vi "dfd_DFXPSimu Casting (scaler).vi"(5 "quantize output? (T)":bool=TRUE, 7 "op params":T2={"source"=0, "is floating?"=FALSE, "o-mode"=enum."Wrap", "q-mode"=enum."Truncation", "wl"=1, "high limit"=0, "low limit"=0, "iwl"=0, "sign?"=TRUE} {"source" items=["Coef a/k"=0, "Coef b/v"=7, "Input"=1, "Output"=2, "Multiplicand"=3, "Product"=4, "Sum"=5, "Delay"=6, "Gain"=8]}, 8 "filtering statistics in":T6(array[cluster]) {"statistics information"."min value" format="%.2f"; "statistics information"."max value" format="%.2f"; "Quantizer Source" items=["Coefficients a/k"=0, "Coefficients b/v"=7, "Input"=1, "Output"=2, "Multiplicand"=3, "Product"=4, "Sum"=5, "Delay"=6]}, 11 "Value in":T7 {"Low 64" format="%.0x"; "High 64" format="%.0x"}) -> (0 "filtering statistics out":T6(array[cluster]) {"statistics information"."min value" format="%.2f"; "statistics information"."max value" format="%.2f"; "Quantizer Source" items=["Coefficients a/k"=0, "Coefficients b/v"=7, "Input"=1, "Output"=2, "Multiplicand"=3, "Product"=4, "Sum"=5, "Delay"=6]}, 3 "Value out":T1={"value"=0, "wl"=0, "iwl"=0, "Signed"=TRUE} {"value" format="%.0x"})   [LabVIEW 2017, in "NI_DigFilter_FXP.lvlib"]
uses:
  <vilib>/addons/Digital Filter Design/NI_DigFilter_FXP.lvlib
  <vilib>/addons/Digital Filter Design/_Objects.llb/dfd_DFXP Data Type 128bits (scaler).ctl
  <vilib>/addons/Digital Filter Design/_Objects.llb/dfd_DFXP Data Type (scaler).ctl
  <vilib>/addons/Digital Filter Design/_Objects.llb/DFD Quantization Sources.ctl
  <vilib>/addons/Digital Filter Design/_Objects.llb/DFD FXP Statistics Data.ctl
  <vilib>/addons/Digital Filter Design/_Objects.llb/dfd_DFXP Operation Parameter.ctl
  <vilib>/addons/Digital Filter Design/_Objects.llb/dfd_Internal Quantization Srcs.ctl
  <vilib>/addons/Digital Filter Design/NI_DigFilterLicensed.lvlib
panel:
  in  "Value out type":T1={"value"=0, "wl"=0, "iwl"=0, "Signed"=TRUE} {"value" format="%.0x"}
  in  "Value out type":T1={"value"=0, "wl"=0, "iwl"=0, "Signed"=TRUE} {"value" format="%.0x"}
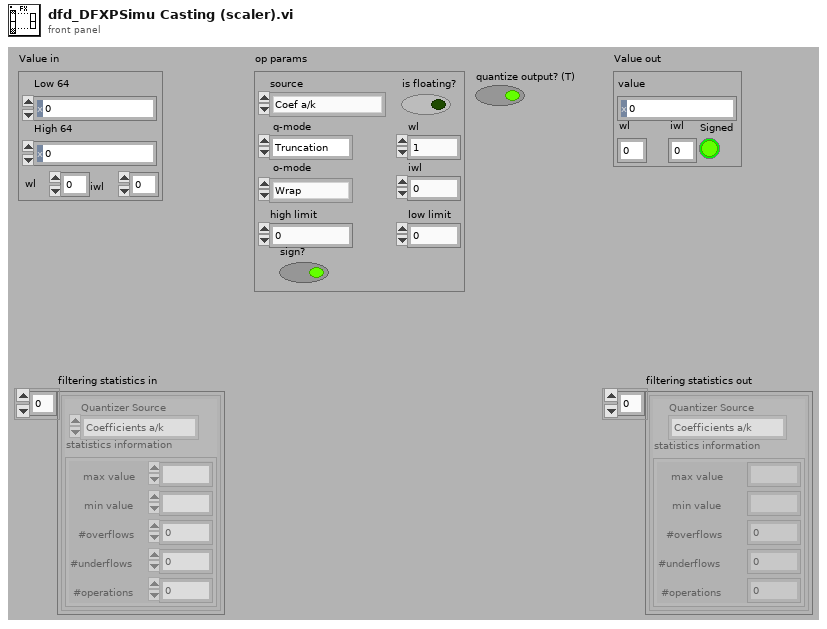
[diagram p1: front panel]
types:
  T1 = typedef "dfd_DFXP Data Type (scaler).ctl" = cluster{"value":i64, "wl":i16, "iwl":i16, "Signed":bool}
  T2 = typedef "dfd_DFXP Operation Parameter.ctl" = cluster{"source":T3, "is floating?":bool, "o-mode":enum16{"Saturation", "Wrap"}, "q-mode":enum16{"Nearest", "Truncation"}, "wl":i16, "high limit":i64, "low limit":i64, "iwl":i16, "sign?":bool}
  T3 = typedef "NI_DigFilterLicensed.lvlib/dfd_Internal Quantization Srcs.ctl" = u16
  T4 = typedef "NI_DigFilterLicensed.lvlib/DFD Quantization Sources.ctl" = u16
  T5 = typedef "NI_DigFilterLicensed.lvlib/DFD FXP Statistics Data.ctl" = cluster{"max value":ext, "min value":ext, "#overflows":i32, "#underflows":i32, "#operations":i32}
  T6 = cluster{"Quantizer Source":T4, "statistics information":T5}[]
  T7 = typedef "dfd_DFXP Data Type 128bits (scaler).ctl" = cluster{"Low 64":u64, "High 64":i64, "wl":i16, "iwl":i16}
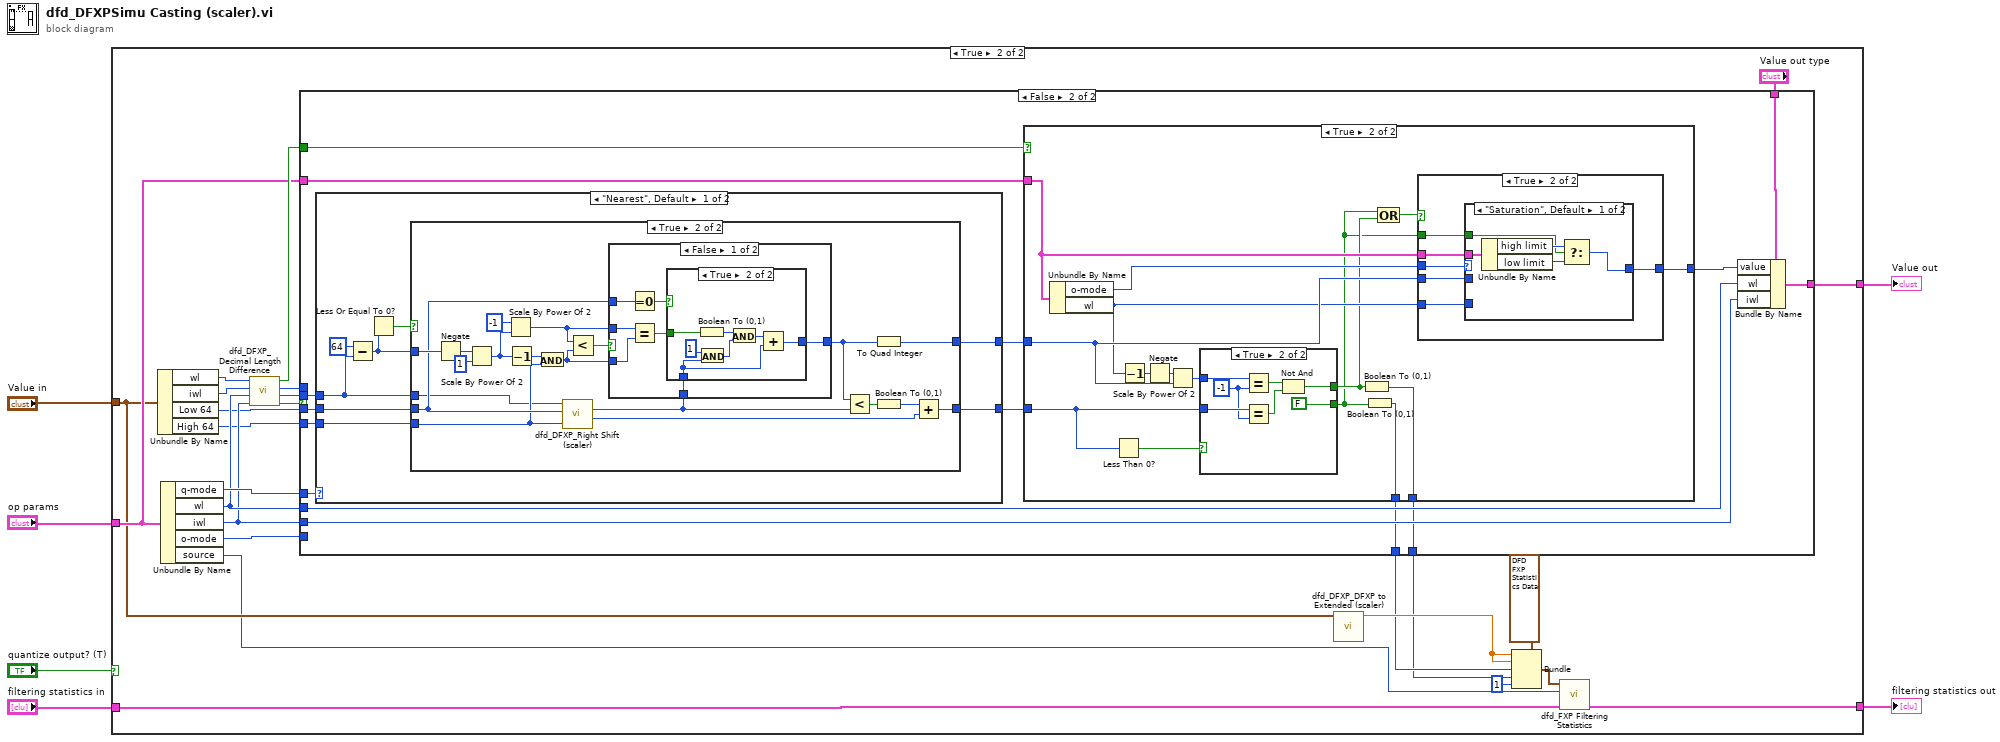
[diagram p0: block diagram]
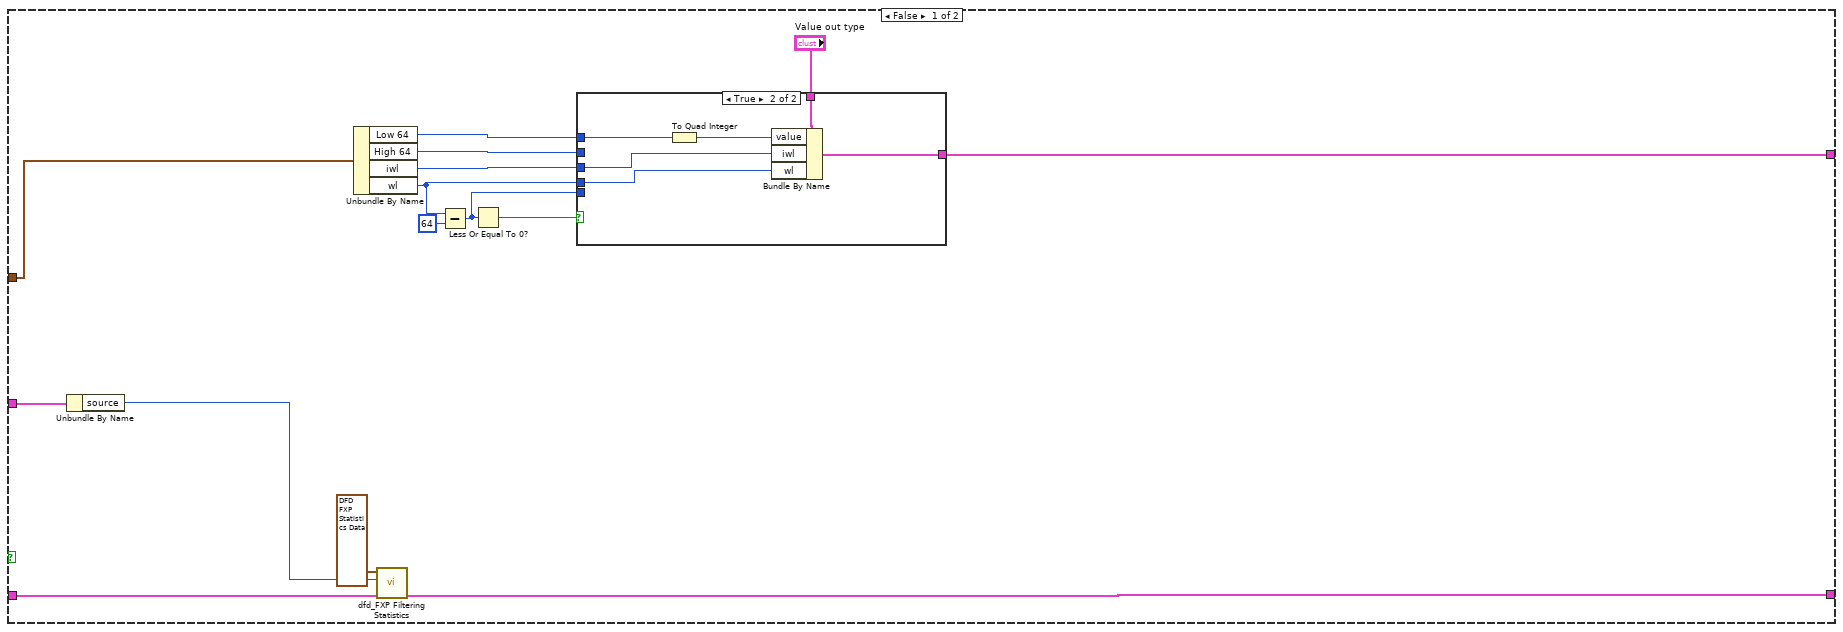
[diagram p2: hidden frame]
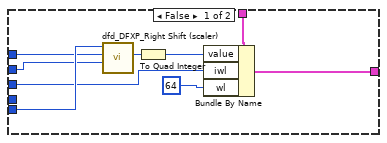
[diagram p3: hidden frame]
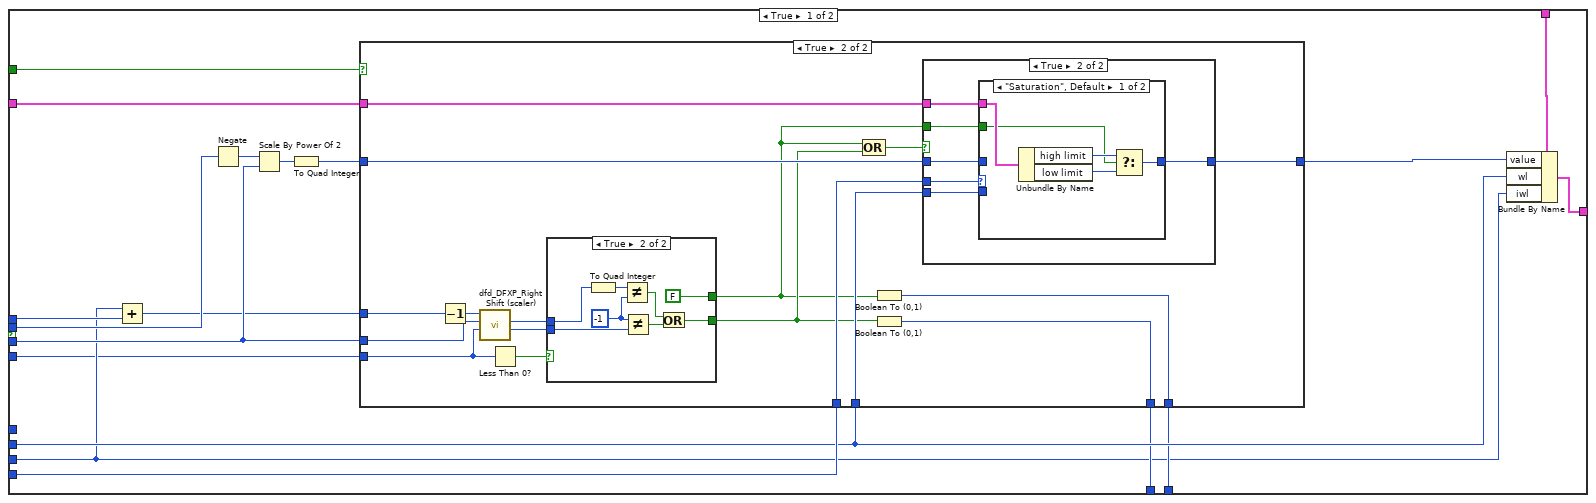
[diagram p4: hidden frame]
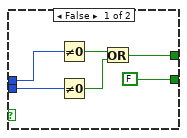
[diagram p6: hidden frame]
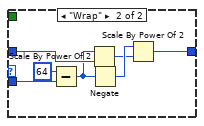
[diagram p8: hidden frame]
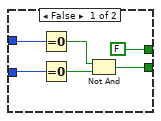
[diagram p10: hidden frame]
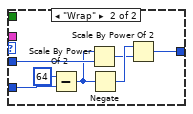
[diagram p12: hidden frame]
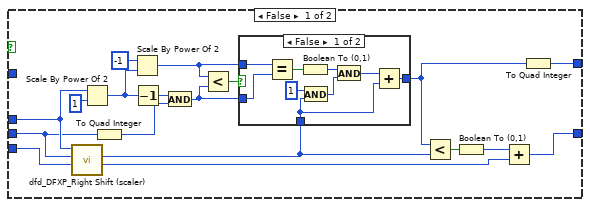
[diagram p13: hidden frame]
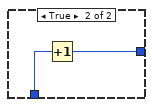
[diagram p14: hidden frame]
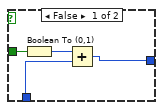
[diagram p15: hidden frame]
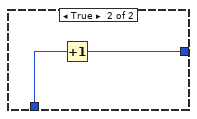
[diagram p16: hidden frame]
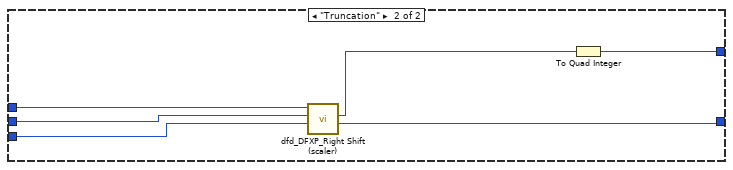
[diagram p17: hidden frame]
diagram:
  n1 = case shown="True" "quantize output? (T)" {
    tunnel: [w12 w50] -> w1
    tunnel: "op params" -> [w21 w53]
    tunnel: "Value in" -> [w13 w46]
    tunnel: "filtering statistics in" -> [w8 w39]
    tunnel: [w7 w38] -> w2
    frame False {
      n2 = Unbundle By Name(w21) -> ("source"=w10:T3)
      n3 = Unbundle By Name(w13) -> ("Low 64"=w19:u64, "High 64"=w17:i64, "iwl"=w18:i16, "wl"=w15:i16)
      n4 = call <vilib>:"dfd_FXP Filtering Statistics.vi"("filtering statistics in"=w8, "source"=w10, "new data"=T5 {"max value"=-inf, "min value"=inf, "#overflows"=0, "#underflows"=0, "#operations"=1}) -> ("filtering statistics out"=w7:T6)  [unwired: 8 in]
      n5 = Subtract(x=w15, y=i16 64) -> (x-y=w16:i16)
      n6 = Less Or Equal To 0?(x=w16) -> (x <= 0?=w11:bool)
      n7 = case shown="True" w11 {
        tunnel: w19 -> [w29 w36]
        tunnel: w18 -> [w25 w34]
        tunnel: [w23 w33] -> w12
        tunnel: w17 -> [w28 _]
        tunnel: w16 -> [w30 _]
        tunnel: w15 -> [_ w32]
        tunnel: "Value out type" -> [w22 w31]
        frame False {
          n8 = call <vilib>:"dfd_DFXP_Right Shift (scaler).vi"("High 64"=w28, "Low 64"=w29, "Num"=w30) -> ("Low 64"=w26:u64)  [unwired: 8 out]
          n9 = To Quad Integer(1:w26) -> (0:w27:i64)
          n10 = Bundle By Name(cluster=w22, "value"=w27, "iwl"=w25, "wl"=i16 64) -> (w23:T1)
        }
        frame True {
          n11 = To Quad Integer(1:w36) -> (0:w35:i64)
          n12 = Bundle By Name(cluster=w31, "value"=w35, "iwl"=w34, "wl"=w32) -> (w33:T1)
        }
      }
    }
    frame True {
      n13 = Unbundle By Name(w46) -> ("wl"=w59:i16, "iwl"=w60:i16, "Low 64"=w49:u64, "High 64"=w48:i64)
      n14 = Unbundle By Name(w53) -> ("q-mode"=w61:enum16{"Nearest", "Truncation"}, "wl"=w54:i16, "iwl"=w52:i16, "o-mode"=w55:enum16{"Saturation", "Wrap"}, "source"=w40:T3)
      n15 = call <vilib>:"dfd_DFXP_Decimal Length Difference.vi"("iwl 2"=w52, "wl 2"=w54, "iwl 1"=w60, "wl 1"=w59) -> ("fwl_diff <= 0?"=w58:bool, "fwl_diff"=w56:i16, "fwl"=w47:i16, "iwl_diff >= 0?"=w57:bool)  [unwired: 4 out]
      n16 = case shown="False" w58 {
        tunnel: w61 -> [_ w145]
        tunnel: w49 -> [w70 w144]
        tunnel: w53 -> [w78 w140]
        tunnel: w57 -> [w71 w142]
        tunnel: w56 -> [w69 w141]
        tunnel: w55 -> [w77 _]
        tunnel: w54 -> [w73 w137]
        tunnel: [w72 w135] -> w50
        tunnel: w52 -> [w64 w136]
        tunnel: "Value out type" -> [w75 w139]
        tunnel: [w68 w134] -> w43
        tunnel: [w67 w133] -> w42
        tunnel: w48 -> [w62 w132]
        tunnel: w47 -> [w65 _]
        frame True {
          n17 = Add(x=w64, y=w65) -> (x+y=w63:i16)
          n18 = Negate(x=w69) -> (-x=w79:i16)
          n19 = Scale By Power Of 2(n=w79, x=w70) -> (x*2^n=w76:u64)
          n20 = To Quad Integer(1:w76) -> (0:w66:i64)
          n21 = case shown="True" w71 {
            tunnel: w78 -> [_ w96]
            tunnel: w77 -> [_ w95]
            tunnel: w66 -> [w80 w94]
            tunnel: [w80 w93] -> w74
            tunnel: w73 -> [_ w92]
            tunnel: w70 -> [_ w88]
            tunnel: [_ w90] -> w68
            tunnel: [_ w91] -> w67
            tunnel: w63 -> [_ w89]
            tunnel: w62 -> [_ w81]
            frame False {
            }
            frame True {
              n22 = Decrement(x=w89) -> (x-1=w85:i16)
              n23 = call <vilib>:"dfd_DFXP_Right Shift (scaler).vi"("High 64"=w81, "Low 64"=w88, "Num"=w85) -> ("High 64"=w86:i64, "Low 64"=w87:u64)  [unwired: 7 out]
              n24 = Less Than 0?(x=w81) -> (x < 0?=w84:bool)
              n25 = case shown="True" w84 {
                tunnel: [w100 FALSE] -> w82
                tunnel: [FALSE w111] -> w83
                tunnel: w87 -> [w102 w107]
                tunnel: w86 -> [w101 w106]
                frame False {
                  n26 = Not Equal To 0?(x=w102) -> (x != 0?=w99:bool)
                  n27 = Not Equal To 0?(x=w101) -> (x != 0?=w98:bool)
                  n28 = Or(x=w99, y=w98) -> (x .or. y?=w100:bool)
                }
                frame True {
                  w109 = i64 -1 ("y")
                  n29 = To Quad Integer(1:w107) -> (0:w105:i64)
                  n30 = Not Equal?(x=w105, y=w109) -> (x != y?=w110:bool)
                  n31 = Not Equal?(x=w109, y=w106) -> (x != y?=w108:bool)
                  n32 = Or(x=w110, y=w108) -> (x .or. y?=w111:bool)
                }
              }
              n33 = Compound Arithmetic op=OR(w82, w83) -> (w97:bool)
              n34 = Boolean To (0,1)(Boolean=w82) -> (0, 1=w91:i16)
              n35 = Boolean To (0,1)(Boolean=w83) -> (0, 1=w90:i16)
              n36 = case shown="True" w97 {
                tunnel: w95 -> [_ w118]
                tunnel: [w112 w117] -> w93
                tunnel: w92 -> [_ w116]
                tunnel: w94 -> [w112 w115]
                tunnel: w96 -> [_ w114]
                tunnel: w82 -> [_ w113]
                frame False {
                }
                frame True {
                  n37 = case shown="\"Saturation\", Default" w118 {
                    tunnel: [w120 w129] -> w117
                    tunnel: w116 -> [_ w130]
                    tunnel: w115 -> [_ w128]
                    tunnel: w114 -> [w123 _]
                    tunnel: w113 -> [w119 _]
                    frame "Saturation", Default {
                      n38 = Unbundle By Name(w123) -> ("high limit"=w122:i64, "low limit"=w121:i64)
                      n39 = Select(t=w122, s=w119, f=w121) -> (s? t:f=w120:i64)
                    }
                    frame "Wrap" {
                      n40 = Subtract(x=i16 64, y=w130) -> (x-y=w126:i16)
                      n41 = Scale By Power Of 2(n=w126, x=w128) -> (x*2^n=w124:i64)
                      n42 = Negate(x=w126) -> (-x=w125:i16)
                      n43 = Scale By Power Of 2(n=w125, x=w124) -> (x*2^n=w129:i64)
                    }
                  }
                }
              }
            }
          }
          n44 = Bundle By Name(cluster=w75, "value"=w74, "wl"=w73, "iwl"=w64) -> (w72:T1)
        }
        frame False {
          n45 = case shown="\"Nearest\", Default" w145 {
            tunnel: w141 -> [w199 w275]
            tunnel: w144 -> [w200 w274]
            tunnel: [w198 w270] -> w143
            tunnel: w132 -> [w197 w273]
            tunnel: [w194 w271] -> w131
            frame "Nearest", Default {
              n46 = Subtract(x=i16 64 ("y"), y=w199) -> (x-y=w195:i16)
              n47 = Less Or Equal To 0?(x=w195) -> (x <= 0?=w196:bool)
              n48 = case shown="True" w196 {
                tunnel: w200 -> [w211 w240]
                tunnel: w199 -> [w212 w238]
                tunnel: [w202 w231] -> w198
                tunnel: w197 -> [w210 w239]
                tunnel: w195 -> [_ w242]
                tunnel: [w204 w232] -> w194
                frame False {
                  n49 = call <vilib>:"dfd_DFXP_Right Shift (scaler).vi"("High 64"=w210, "Low 64"=w211, "Num"=w212) -> ("High 64"=w205:i64, "Low 64"=w208:u64)  [unwired: 7 out]
                  n50 = Scale By Power Of 2(n=w212, x=i64 1) -> (x*2^n=w216:i64)
                  n51 = To Quad Integer(1:w211) -> (0:w209:i64)
                  n52 = Scale By Power Of 2(n=-1, x=w216) -> (x*2^n=w217:i64)
                  n53 = Decrement(x=w216) -> (x-1=w214:i64)
                  n54 = And(x=w214, y=w209) -> (x .and. y?=w218:i64)
                  n55 = Less?(x=w217, y=w218) -> (x < y?=w219:bool)
                  n56 = case shown="False" w219 {
                    tunnel: w217 -> [w228 _]
                    tunnel: w218 -> [w227 _]
                    tunnel: w208 -> [w220 w230]
                    tunnel: [w222 w229] -> w203
                    frame False {
                      n57 = Equal?(x=w228, y=w227) -> (x = y?=w225:bool)
                      n58 = Boolean To (0,1)(Boolean=w225) -> (0, 1=w224:i16)
                      n59 = And(x=u64 1, y=w220) -> (x .and. y?=w223:u64)
                      n60 = And(x=w224, y=w223) -> (x .and. y?=w221:u64)
                      n61 = Add(x=w221, y=w220) -> (x+y=w222:u64)
                    }
                    frame True {
                      n62 = Increment(x=w230) -> (x+1=w229:u64)
                    }
                  }
                  n63 = Less?(x=w203, y=w208) -> (x < y?=w207:bool)
                  n64 = Boolean To (0,1)(Boolean=w207) -> (0, 1=w206:i16)
                  n65 = Add(x=w206, y=w205) -> (x+y=w204:i64)
                  n66 = To Quad Integer(1:w203) -> (0:w202:i64)
                }
                frame True {
                  n67 = Negate(x=w242) -> (-x=w241:i16)
                  n68 = Scale By Power Of 2(n=w241, x=i64 1) -> (x*2^n=w246:i64)
                  n69 = Scale By Power Of 2(n=-1, x=w246) -> (x*2^n=w245:i64)
                  n70 = Decrement(x=w246) -> (x-1=w248:i64)
                  n71 = And(x=w248, y=w239) -> (x .and. y?=w244:i64)
                  n72 = call <vilib>:"dfd_DFXP_Right Shift (scaler).vi"("High 64"=w239, "Low 64"=w240, "Num"=w238) -> ("High 64"=w233:i64, "Low 64"=w236:u64)  [unwired: 7 out]
                  n73 = Less?(x=w245, y=w244) -> (x < y?=w243:bool)
                  n74 = case shown="False" w243 {
                    tunnel: w245 -> [w256 _]
                    tunnel: w244 -> [w255 _]
                    tunnel: w236 -> [w251 w269]
                    tunnel: [w250 w268] -> w237
                    tunnel: w240 -> [w254 _]
                    frame False {
                      n75 = Equal To 0?(x=w254) -> (x = 0?=w253:bool)
                      n76 = Equal?(x=w256, y=w255) -> (x = y?=w252:bool)
                      n77 = case shown="True" w253 {
                        tunnel: w252 -> [w260 w263]
                        tunnel: w251 -> [w258 w262]
                        tunnel: [w257 w261] -> w250
                        frame False {
                          n78 = Boolean To (0,1)(Boolean=w260) -> (0, 1=w259:i16)
                          n79 = Add(x=w259, y=w258) -> (x+y=w257:u64)
                        }
                        frame True {
                          n80 = Boolean To (0,1)(Boolean=w263) -> (0, 1=w265:i16)
                          n81 = And(x=u64 1, y=w262) -> (x .and. y?=w266:u64)
                          n82 = And(x=w265, y=w266) -> (x .and. y?=w267:u64)
                          n83 = Add(x=w267, y=w262) -> (x+y=w261:u64)
                        }
                      }
                    }
                    frame True {
                      n84 = Increment(x=w269) -> (x+1=w268:u64)
                    }
                  }
                  n85 = Less?(x=w237, y=w236) -> (x < y?=w235:bool)
                  n86 = To Quad Integer(1:w237) -> (0:w231:i64)
                  n87 = Boolean To (0,1)(Boolean=w235) -> (0, 1=w234:i16)
                  n88 = Add(x=w234, y=w233) -> (x+y=w232:i64)
                }
              }
            }
            frame "Truncation" {
              n89 = call <vilib>:"dfd_DFXP_Right Shift (scaler).vi"("High 64"=w273, "Low 64"=w274, "Num"=w275) -> ("High 64"=w271:i64, "Low 64"=w272:u64)  [unwired: 7 out]
              n90 = To Quad Integer(1:w272) -> (0:w270:i64)
            }
          }
          n91 = case shown="True" w142 {
            tunnel: w143 -> [w146 w155]
            tunnel: w140 -> [_ w159]
            tunnel: [w146 w158] -> w138
            tunnel: [_ w156] -> w134
            tunnel: [_ w157] -> w133
            tunnel: w131 -> [_ w150]
            frame False {
            }
            frame True {
              n92 = Unbundle By Name(w159) -> ("o-mode"=w160:enum16{"Saturation", "Wrap"}, "wl"=w154:i16)
              n93 = Less Than 0?(x=w150) -> (x < 0?=w152:bool)
              n94 = Decrement(x=w154) -> (x-1=w147:i16)
              n95 = Negate(x=w147) -> (-x=w153:i16)
              n96 = Scale By Power Of 2(n=w153, x=w155) -> (x*2^n=w151:i64)
              n97 = case shown="True" w152 {
                tunnel: w151 -> [w167 w174]
                tunnel: w150 -> [w166 w173]
                tunnel: [FALSE w169] -> w149
                tunnel: [w163 FALSE (".not. (x .and. y)?")] -> w148
                frame False {
                  n98 = Equal To 0?(x=w167) -> (x = 0?=w164:bool)
                  n99 = Equal To 0?(x=w166) -> (x = 0?=w165:bool)
                  n100 = Not And(1:w165, 2:w164) -> (0:w163:bool)
                }
                frame True {
                  w172 = i64 -1 ("y")
                  n101 = Equal?(x=w174, y=w172) -> (x = y?=w171:bool)
                  n102 = Equal?(x=w173, y=w172) -> (x = y?=w170:bool)
                  n103 = Not And(1:w170, 2:w171) -> (0:w169:bool)
                }
              }
              n104 = Boolean To (0,1)(Boolean=w149) -> (0, 1=w157:i16)
              n105 = Boolean To (0,1)(Boolean=w148) -> (0, 1=w156:i16)
              n106 = Compound Arithmetic op=OR(w148, w149) -> (w161:bool)
              n107 = case shown="True" w161 {
                tunnel: w160 -> [_ w181]
                tunnel: [w175 w180] -> w158
                tunnel: w154 -> [_ w179]
                tunnel: w155 -> [w175 w178]
                tunnel: w159 -> [_ w177]
                tunnel: w148 -> [_ w176]
                frame False {
                }
                frame True {
                  n108 = case shown="\"Saturation\", Default" w181 {
                    tunnel: [w183 w192] -> w180
                    tunnel: w179 -> [_ w193]
                    tunnel: w178 -> [_ w191]
                    tunnel: w177 -> [w186 _]
                    tunnel: w176 -> [w182 _]
                    frame "Saturation", Default {
                      n109 = Unbundle By Name(w186) -> ("high limit"=w185:i64, "low limit"=w184:i64)
                      n110 = Select(t=w185, s=w182, f=w184) -> (s? t:f=w183:i64)
                    }
                    frame "Wrap" {
                      n111 = Subtract(x=i16 64, y=w193) -> (x-y=w189:i16)
                      n112 = Scale By Power Of 2(n=w189, x=w191) -> (x*2^n=w187:i64)
                      n113 = Negate(x=w189) -> (-x=w188:i16)
                      n114 = Scale By Power Of 2(n=w188, x=w187) -> (x*2^n=w192:i64)
                    }
                  }
                }
              }
            }
          }
          n115 = Bundle By Name(cluster=w139, "value"=w138, "wl"=w137, "iwl"=w136) -> (w135:T1)
        }
      }
      n116 = call <vilib>:"dfd_DFXP_DFXP to Extended (scaler).vi"("Value in"=w46) -> ("Ext value"=w44:ext)  [unwired: 10 out]
      n117 = Bundle(cluster=T5 {"max value"=-inf, "min value"=inf, "#overflows"=0, "#underflows"=0, "#operations"=1} ("new data"), "max value"=w44, "min value"=w44, "#overflows"=w43, "#underflows"=w42, "#operations"=1) -> (w41:T5)
      n118 = call <vilib>:"dfd_FXP Filtering Statistics.vi"("filtering statistics in"=w39, "source"=w40, "new data"=w41) -> ("filtering statistics out"=w38:T6)  [unwired: 8 in]
    }
  }
  "Value out" <- w1
  "filtering statistics out" <- w2
